vi "translatePolarityValues.vi"(0 "ACESDEController in":refnum<class "ACESDEController.lvclass">, 1 "simple_actions":T3, 2 "polarity_value(s) (in)":u32, 3 "polarity_items (in)":T1[](array[typedef]), 5 "error in (no error)":errorcluster) -> (14 "ACESDEController out":refnum<class "ACESDEController.lvclass">, 16 "polarity_value (out)":u32, 17 "polarity_items (out)":T1[](array[typedef]), 19 "error out":errorcluster)   [LabVIEW 2020, in "classes.lvlib" / "ACESDEController.lvclass"]
uses:
  ACESDEController.lvclass
  simple_actions.ctl
  polarity_item.ctl
  polarity.ctl
  common.lvlib
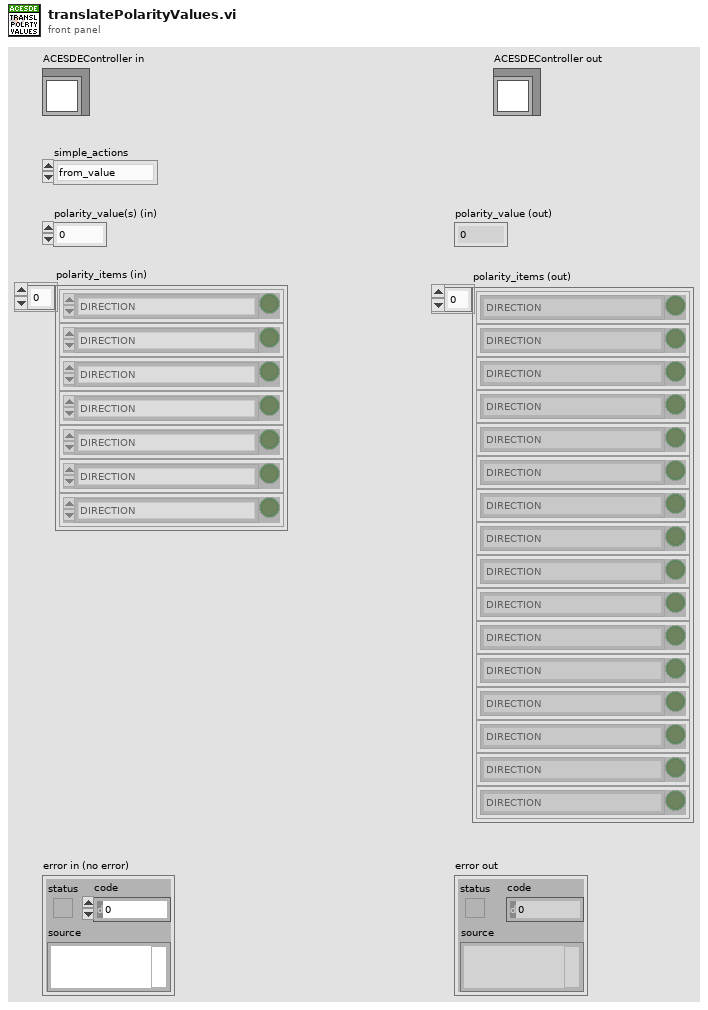
[diagram p1: front panel]
types:
  T1 = typedef "common.lvlib/polarity_item.ctl" = cluster{"item":T2, "status":bool}
  T2 = typedef "common.lvlib/polarity.ctl" = enum16{"DIRECTION", "LIMIT", "HOME", "DIG_OUT", "DIG_IN", "ENABLE_OUT", "JUMP_ERR", "LATCH", "Z-CHAN_INDEX", "ENCODER_DECODING:1X", "ENCODER_DECODING:2X", "ENCODER_DECODING:4X", "ALARM", "STANDALONE_ERR", "-", "<reserved/nc>"}
  T3 = typedef "common.lvlib/simple_actions.ctl" = enum16{"from_value", "to_value"}
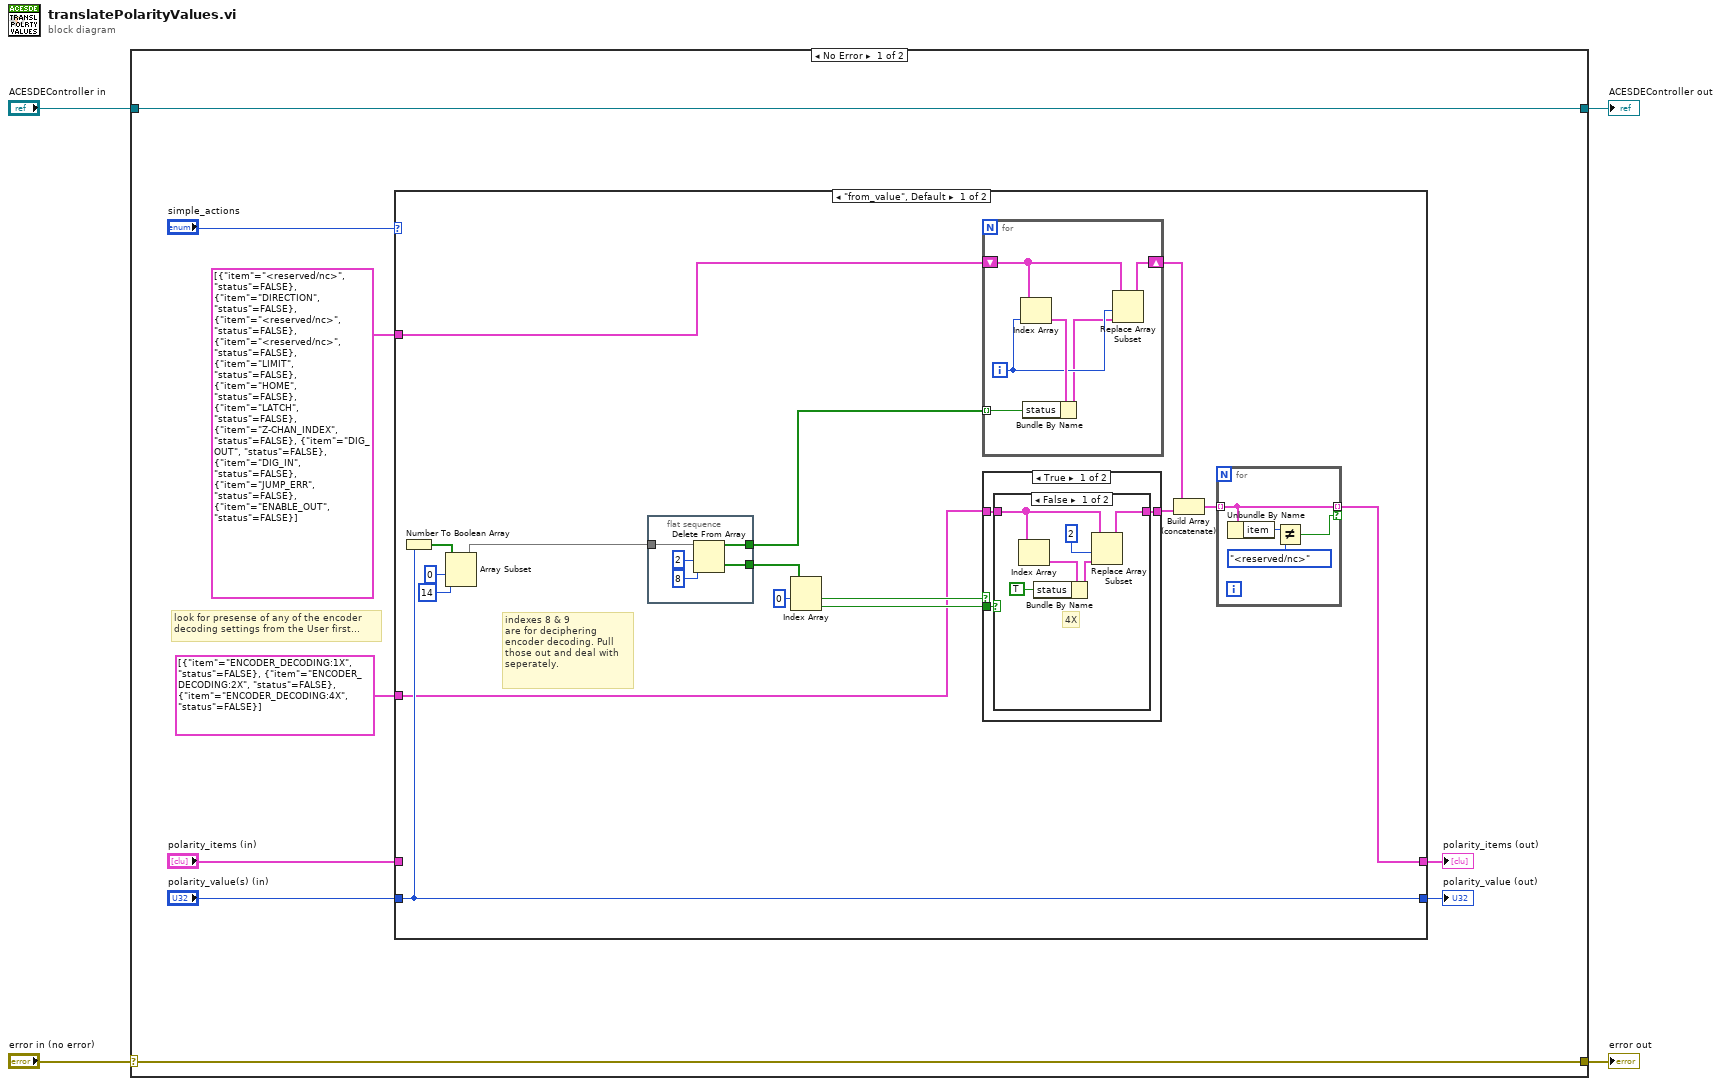
[diagram p0: block diagram]
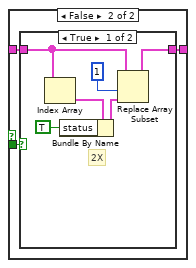
[diagram p3: hidden frame]
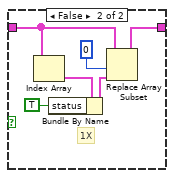
[diagram p4: hidden frame]
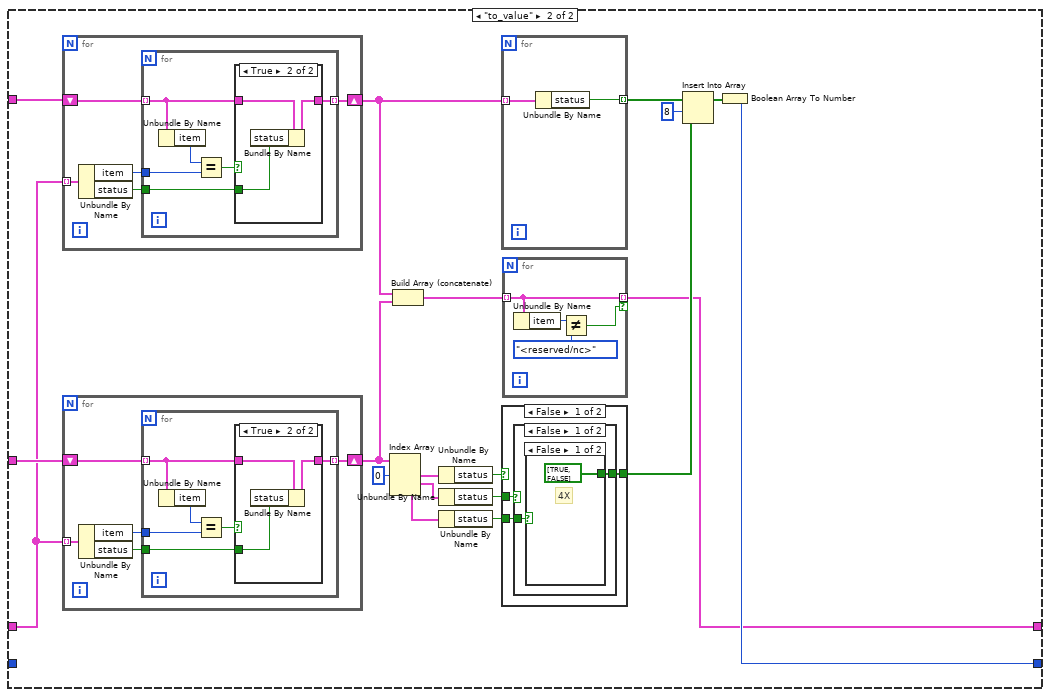
[diagram p5: hidden frame]
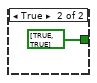
[diagram p7: hidden frame]
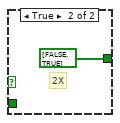
[diagram p8: hidden frame]
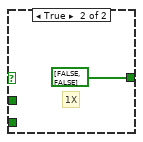
[diagram p9: hidden frame]
diagram:
  n1 = case shown="No Error" "error in (no error)" {
    selector: "error in (no error)" -> [w12 w135]
    tunnel: [w12 w135] -> w3
    tunnel: [w13 w134] -> w1
    tunnel: "ACESDEController in" -> [w13 w134]
    frame No Error {
      # "look for presense of any of the encoder\ndecoding settings from the User first..."
      n2 = case shown="\"from_value\", Default" "simple_actions" {
        tunnel: "polarity_value(s) (in)" -> [w25 _]
        tunnel: [w14 w70] -> w9
        tunnel: T1[] [{"item"=enum."<reserved/nc>", "status"=FALSE}, {"item"=enum."DIRECTION", "status"=FALSE}, {"item"=enum."<reserved/nc>", "status"=FALSE}, {"item"=enum."<reserved/nc>", "status"=FALSE}, {"item"=enum."LIMIT", "status"=FALSE}, {"item"=enum."HOME", "status"=FALSE}, {"item"=enum."LATCH", "status"=FALSE}, {"item"=enum."Z-CHAN_INDEX", "status"=FALSE}, {"item"=enum."DIG_OUT", "status"=FALSE}, {"item"=enum."DIG_IN", "status"=FALSE}, {"item"=enum."JUMP_ERR", "status"=FALSE}, {"item"=enum."ENABLE_OUT", "status"=FALSE}] ("polarity_items (in)") -> [w26 w80]
        tunnel: "polarity_items (in)" -> [_ w74]
        tunnel: [w25 w72] -> w6
        tunnel: T1[] [{"item"=enum."ENCODER_DECODING:1X", "status"=FALSE}, {"item"=enum."ENCODER_DECODING:2X", "status"=FALSE}, {"item"=enum."ENCODER_DECODING:4X", "status"=FALSE}] -> [w17 w88]
        frame "from_value", Default {
          # "indexes 8 & 9 \nare for deciphering\nencoder decoding. Pull\nthose out and deal with \nseperately."
          n3 = Number To Boolean Array(number=w25) -> (Boolean array=w29:bool[])
          n4 = Array Subset(array=w29, index=0, length=14) -> (w16:bool[])
          n5 = flat-sequence {
            tunnel: w16 -> [w63]
            tunnel: [w60] -> w24
            tunnel: [w59] -> w23
            frame #0 {
              n6 = Delete From Array(array=w63, length=2 ("index"), index=8) -> (deleted portion=w59:bool[], array with subset deleted=w60:bool[])
            }
          }
          n7 = Index Array(array=w23, index #1=0 ("index")) -> (element #1=w21:bool, element #2=w20:bool)  [unwired: 1 in]
          n8 = for {
            shift-right: [w64] -> w19
            shift-left: w26 -> [w67]
            tunnel: w24 -> [w68] mode=indexing
            i -> [w66]
            n9 = Index Array(array=w67, index=w66) -> (element=w69:T1)
            n10 = Bundle By Name(cluster=w69, "status"=w68) -> (w65:T1)
            n11 = Replace Array Subset(array=w67, new element=w65, index=w66) -> (w64:T1[])
          }
          n12 = case shown="True" w21 {
            tunnel: w20 -> [w36 w46]
            tunnel: w17 -> [w35 w45]
            tunnel: [w34 w44] -> w18
            frame True {
              n13 = case shown="False" w36 {
                tunnel: w35 -> [w37 w43]
                tunnel: [w38 w43] -> w34
                frame False {
                  # "4X"
                  n14 = Index Array(array=w37) -> (element=w41:T1)  [unwired: 1 in]
                  n15 = Bundle By Name(cluster=w41, "status"=TRUE) -> (w42:T1)
                  n16 = Replace Array Subset(array=w37, new element=w42, index=2) -> (w38:T1[])
                }
                frame True {
                }
              }
            }
            frame False {
              n17 = case shown="True" w46 {
                tunnel: w45 -> [w47 w53]
                tunnel: [w48 w54] -> w44
                frame True {
                  # "2X"
                  n18 = Index Array(array=w47) -> (element=w51:T1)  [unwired: 1 in]
                  n19 = Bundle By Name(cluster=w51, "status"=TRUE) -> (w52:T1)
                  n20 = Replace Array Subset(array=w47, new element=w52, index=1) -> (w48:T1[])
                }
                frame False {
                  # "1X"
                  n21 = Index Array(array=w53) -> (element=w57:T1)  [unwired: 1 in]
                  n22 = Bundle By Name(cluster=w57, "status"=TRUE) -> (w58:T1)
                  n23 = Replace Array Subset(array=w53, new element=w58, index=0) -> (w54:T1[])
                }
              }
            }
          }
          n24 = Build Array (concatenate)(w19, w18) -> (w15:T1[])
          n25 = for {
            tunnel: w15 -> [w30] mode=indexing
            tunnel: [w30] -> w14 mode=indexing if=w31
            n26 = Unbundle By Name(w30) -> ("item"=w33:T2)
            n27 = Not Equal?(x=w33, y=polarity."<reserved/nc>" ("item")) -> (x != y?=w31:bool)
          }
        }
        frame "to_value" {
          n28 = for {
            shift-right: [w95] -> w76
            shift-left: w80 -> [w98]
            tunnel: w74 -> [w99] mode=indexing
            n29 = Unbundle By Name(w99) -> ("item"=w97:T2, "status"=w96:bool)
            n30 = for {
              tunnel: w98 -> [w102] mode=indexing
              tunnel: w97 -> [w104]
              tunnel: w96 -> [w101]
              tunnel: [w100] -> w95 mode=indexing
              n31 = Unbundle By Name(w102) -> ("item"=w105:T2)
              n32 = Equal?(x=w105, y=w104) -> (x = y?=w103:bool)
              n33 = case shown="True" w103 {
                tunnel: w102 -> [w106 w109]
                tunnel: w101 -> [_ w108]
                tunnel: [w106 w107] -> w100
                frame False {
                }
                frame True {
                  n34 = Bundle By Name(cluster=w109, "status"=w108) -> (w107:T1)
                }
              }
            }
          }
          n35 = for {
            shift-right: [w119] -> w75
            shift-left: w88 -> [w122]
            tunnel: w74 -> [w123] mode=indexing
            n36 = Unbundle By Name(w123) -> ("item"=w121:T2, "status"=w120:bool)
            n37 = for {
              tunnel: w122 -> [w126] mode=indexing
              tunnel: w121 -> [w128]
              tunnel: w120 -> [w125]
              tunnel: [w124] -> w119 mode=indexing
              n38 = Unbundle By Name(w126) -> ("item"=w129:T2)
              n39 = Equal?(x=w129, y=w128) -> (x = y?=w127:bool)
              n40 = case shown="True" w127 {
                tunnel: w126 -> [w130 w133]
                tunnel: w125 -> [_ w132]
                tunnel: [w130 w131] -> w124
                frame False {
                }
                frame True {
                  n41 = Bundle By Name(cluster=w133, "status"=w132) -> (w131:T1)
                }
              }
            }
          }
          n42 = Index Array(array=w75, index #1=0 ("index")) -> (element #1=w86:T1, element #2=w85:T1, element #3=w84:T1)  [unwired: 2 in]
          n43 = Build Array (concatenate)(w76, w75) -> (w71:T1[])
          n44 = Unbundle By Name(w86) -> ("status"=w83:bool)
          n45 = Unbundle By Name(w85) -> ("status"=w82:bool)
          n46 = Unbundle By Name(w84) -> ("status"=w81:bool)
          n47 = for {
            tunnel: w76 -> [w94] mode=indexing
            tunnel: [w93] -> w79 mode=indexing
            n48 = Unbundle By Name(w94) -> ("status"=w93:bool)
          }
          n49 = case shown="False" w83 {
            tunnel: w82 -> [w112 _]
            tunnel: w81 -> [w111 _]
            tunnel: [w110 bool[] [FALSE, FALSE]] -> w77
            frame False {
              n50 = case shown="False" w112 {
                tunnel: w111 -> [w114 _]
                tunnel: [w113 bool[] [FALSE, TRUE]] -> w110
                frame False {
                  n51 = case shown="False" w114 {
                    tunnel: [bool[] [TRUE, FALSE] bool[] [TRUE, TRUE]] -> w113
                    frame False {
                      # "4X"
                    }
                    frame True {
                    }
                  }
                }
                frame True {
                  # "2X"
                }
              }
            }
            frame True {
              # "1X"
            }
          }
          n52 = for {
            tunnel: w71 -> [w89] mode=indexing
            tunnel: [w89] -> w70 mode=indexing if=w90
            n53 = Unbundle By Name(w89) -> ("item"=w92:T2)
            n54 = Not Equal?(x=w92, y=polarity."<reserved/nc>" ("item")) -> (x != y?=w90:bool)
          }
          n55 = Insert Into Array(array=w79, index=8, new element=w77) -> (w73:bool[])
          n56 = Boolean Array To Number(Boolean array=w73) -> (number=w72:u32)
        }
      }
      "polarity_items (out)" <- w9
      "polarity_value (out)" <- w6
    }
    frame Error {
    }
  }
  "error out" <- w3
  "ACESDEController out" <- w1
